vi "cali_building LUT.vi"(6 "z插值点数":i32, 7 "method":i32(ring)=1 caption="方法" items=["最近", "双线性", "双三次", "双三次样条"], 9 "array R":dbl[](array[numeric]), 10 "array piezo":dbl[](array[numeric]), 11 "info":T1={"data name"="", "ROI ref"=refnum, "cali ref"=refnum, "参考球？"=FALSE, "LUT"=[], "Cali array"=[], "修正次数"=2, "R_step"=0.4, "sample(quar)"=12}) -> (3 "new info":T1={"data name"="", "ROI ref"=refnum, "cali ref"=refnum, "参考球？"=FALSE, "LUT"=[], "Cali array"=[], "修正次数"=2, "R_step"=0.4, "sample(quar)"=12})   [LabVIEW 2017]
uses:
  control/bead info.ctl
  <vilib>/vision/Image Controls.llb/IMAQ Image.ctl
  <vilib>/gmath/interp.llb/Create Mesh Grid (2D) (x,y arrays).vi
  <vilib>/gmath/interp.llb/Interpolate 2D (2d X,Y).vi
  <vilib>/gmath/NI_Gmath.lvlib
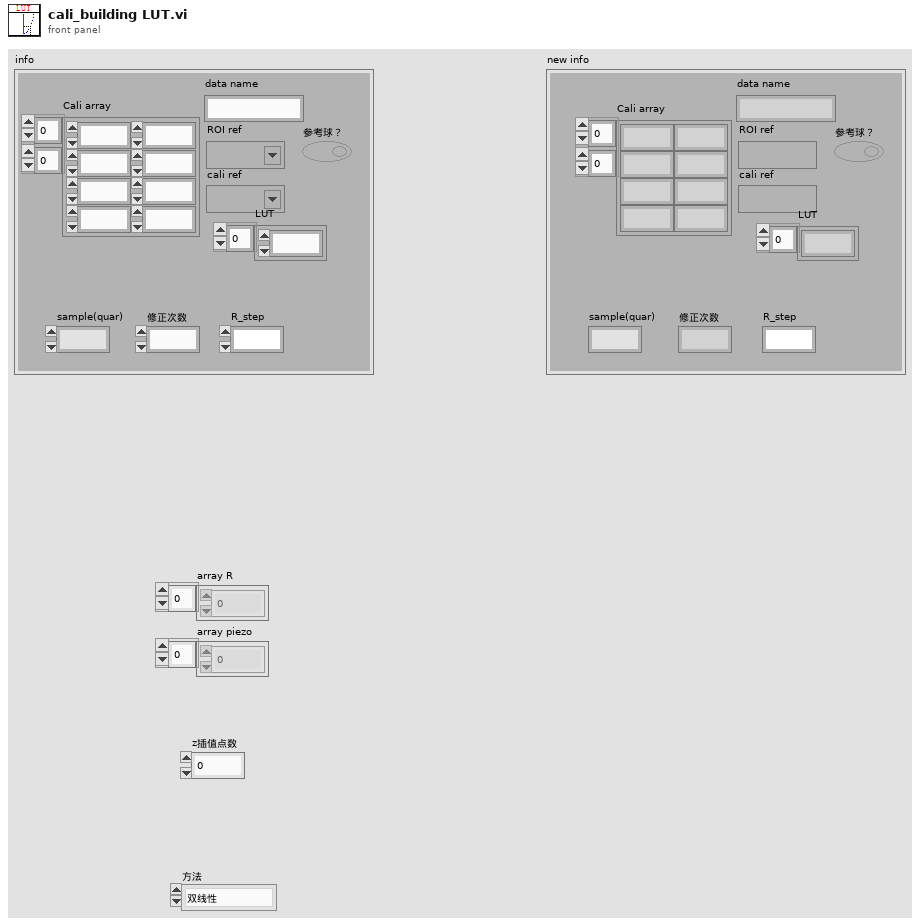
[diagram p1: front panel]
types:
  T1 = typedef "bead info.ctl" = cluster{"data name":string, "ROI ref":T2, "cali ref":T2, "参考球？":bool, "LUT":dbl[], "Cali array":dbl[][], "修正次数":i32, "R_step":dbl, "sample(quar)":i32}
  T2 = typedef "IMAQ Image.ctl" = refnum<image>
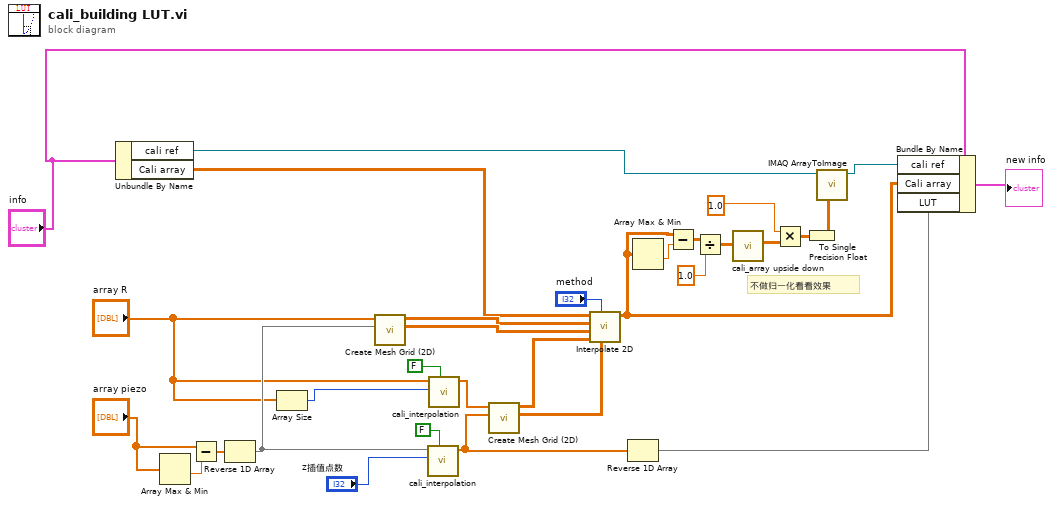
[diagram p0: block diagram]
diagram:
  # "不做归一化看看效果"
  n1 = Unbundle By Name("info") -> ("cali ref"=w12:T2, "Cali array"=w11:dbl[][])
  n2 = Array Max & Min(array="array piezo") -> (min value=w30:dbl)  [unwired: 3 out]
  n3 = Subtract(x="array piezo", y=w30) -> (x-y=w31:dbl[])
  n4 = Reverse 1D Array(array=w31) -> (reversed array=w15:dbl[])
  n5 = Array Size(array="array R") -> (size(s)=w3:i32)
  n6 = call-poly <vilib>:"Create Mesh Grid (2D).vi"("y domain"=w15, "x domain"="array R") -> ("Y"=w24:dbl[][], "X"=w23:dbl[][])  [unwired: 7 in, 1 out]
  n7 = call "cali_interpolation.vi"("降序?"=FALSE, "插值点数"="z插值点数", "array R"=w15) -> ("插值数组"=w13:dbl[])  [unwired: 8 in]
  n8 = call "cali_interpolation.vi"("降序?"=FALSE, "插值点数"=w3, "array R"="array R") -> ("插值数组"=w16:dbl[])  [unwired: 8 in]
  n9 = call-poly <vilib>:"Create Mesh Grid (2D).vi"("y domain"=w13, "x domain"=w16) -> ("Y"=w28:dbl[][], "X"=w27:dbl[][])  [unwired: 7 in, 1 out]
  n10 = call-poly <vilib>:"Interpolate 2D.vi"("yi"=w28, "method"="method", "xi"=w27, "Y"=w24, "X"=w23, "Z"=w11) -> ("zi"=w7:dbl[][])  [unwired: 2 in, 3 out]
  n11 = Reverse 1D Array(array=w13) -> (reversed array=w6:dbl[])
  n12 = Array Max & Min(array=w7) -> (min value=w18:dbl)  [unwired: 3 out]
  n13 = Subtract(x=w7, y=w18) -> (x-y=w19:dbl[][])
  n14 = Divide(x=w19, y=1.0) -> (x/y=w17:dbl[][])
  n15 = call "cali_array upside down.vi"("cali array in"=w17) -> ("cali array out"=w20:dbl[][])  [unwired: 10 in]
  n16 = Multiply(x=1.0, y=w20) -> (x*y=w21:dbl[][])
  n17 = To Single Precision Float(number=w21) -> (single precision float=w22:sgl[][])
  n18 = call "IMAQ ArrayToImage"("Image Pixels (Float)"=w22, "Image"=w12) -> ("Image Out"=w8:T2)  [unwired: 8 in, 1 out]
  n19 = Bundle By Name(cluster="info", "cali ref"=w8, "Cali array"=w7, "LUT"=w6) -> (→"new info":T1)
